vi "Configure Histogram Bin.vi"(6 "Bin Width (0.004)":dbl=0.004, 7 "Bin Count (0)":i32, 8 "error in (no error)":errorcluster, 9 "Center Value (0)":dbl, 10 "Channel (1: Channel 1)":i32(ring)=1 items=["Channel 1"=1, "Channel 2"=2], 11 "VISA resource name":refnum<visa-resource-name>) -> (0 "error out":errorcluster, 3 "VISA resource name out":refnum<visa-resource-name>)   [LabVIEW 2012, in "Keysight B2980 Series.lvlib"]
doc: "Configures the settings of bins for histogram."
uses:
  Keysight B2980 Series.lvlib
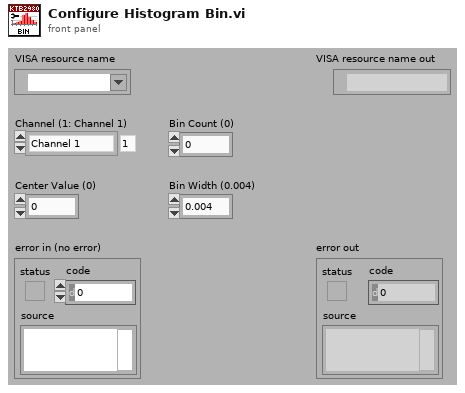
[diagram p1: front panel]
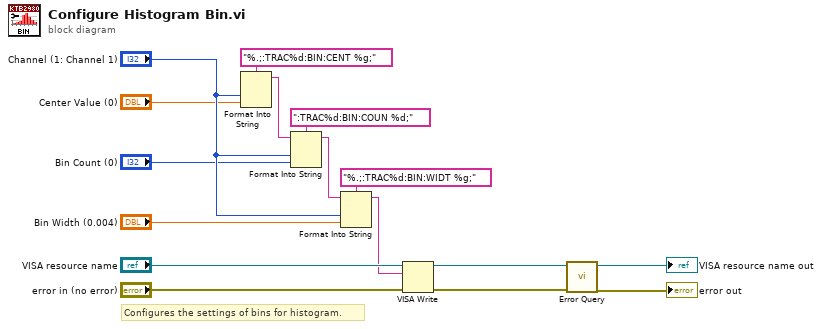
[diagram p0: block diagram]
diagram:
  # "Configures the settings of bins for histogram."
  n1 = Format Into String(format string="%.;:TRAC%d:BIN:CENT %g;", "Channel (1: Channel 1)", "Center Value (0)") -> (resulting string=w13:string)  [unwired: 2 in, 1 out]
  n2 = Format Into String(format string=":TRAC%d:BIN:COUN %d;", initial string=w13, "Channel (1: Channel 1)", "Bin Count (0)") -> (resulting string=w10:string)  [unwired: 1 in, 1 out]
  n3 = Format Into String(format string="%.;:TRAC%d:BIN:WIDT %g;", initial string=w10, "Channel (1: Channel 1)", "Bin Width (0.004)") -> (resulting string=w3:string)  [unwired: 1 in, 1 out]
  n4 = VISA Write(VISA resource name="VISA resource name", write buffer=w3, error in (no error)="error in (no error)") -> (VISA resource name out=w2:refnum<visa-resource-name>, error out=w1:errorcluster)  [unwired: 1 out]
  n5 = call "Error Query.vi"("error in (no error)"=w1, "VISA resource name"=w2) -> ("error out"=→"error out":errorcluster, "VISA resource name out"=→"VISA resource name out":refnum<visa-resource-name>)  [unwired: 8 out]
